vi "InitMiscellaneous.vi"   [LabVIEW 2020]
doc: "This VI initializes miscellaneous devices such as the compressor and any decorations."
uses:
  <vilib>/Rock Robotics/WPI/Compressor/WPI_CompressorFeedbackMode.ctl
  <vilib>/Rock Robotics/SystemInterfaces/DIO/FPGA_DIOPWMChannel.ctl
  refnumbers.vi
  <vilib>/Rock Robotics/WPI/Utilities/WPI_GetSetVariantRefNum.vi
  robotoutputs.vi
types:
  T1 = typedef "FPGA_DIOPWMChannel.ctl" = enum8{"PWM 0", "PWM 1", "PWM 2", "PWM 3", "PWM 4", "PWM 5", "PWM 6", "PWM 7", "PWM 8", "PWM 9", "PWM MXP 0", "PWM MXP 1", "PWM MXP 2", "PWM MXP 3", "PWM MXP 4", "PWM MXP 5", "PWM MXP 6", "PWM MXP 7", "PWM MXP 8", "PWM MXP 9", "Invalid"}
  T2 = typedef "WPI_CompressorFeedbackMode.ctl" = enum16{"Analog Only", "Digital Only", "Hybrid"}
  T3 = cluster{"Feedback Sensor":T2, "Max Pressure (PSI)":dbl, "Min Pressure (PSI)":dbl}
  T4 = typedef "WPI_CompressorDevRef.ctl" = cluster{"DevStatus":errorcluster, "Pneumatics Control Module":u8}
  T5 = typedef "WPI_PWMDeviceRef.ctl" = cluster{"DeviceStatus":errorcluster, "PWM Channel":T1}
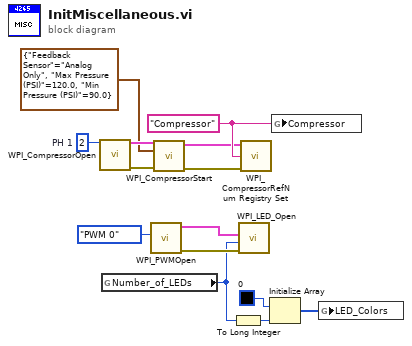
[diagram p0: block diagram]
diagram:
  w11 = "Compressor" ("refnum name")
  w10 = u8 2  # PH 1
  n1 = call <vilib>:"WPI_CompressorOpen.vi"("Pneumatics device (def)"=w10) -> ("CompressorDevRef"=w9:T4, "error out"=w6:errorcluster)  [unwired: 13 in]
  n2 = global read "refnumbers.vi" "Number_of_LEDs"() -> (w1:u16)
  n3 = call <vilib>:"WPI_PWMOpen.vi"("PWM Channel"=FPGA_DIOPWMChannel."PWM 0") -> ("error out"=w3:errorcluster, "PWMDeviceRef"=w4:T5)  [unwired: 9 in]
  n4 = call <vilib>:"WPI_CompressorStart.vi"("error in (no error)"=w6, "Feedback Configuration"=T3 {"Feedback Sensor"=enum."Analog Only", "Max Pressure (PSI)"=120.0, "Min Pressure (PSI)"=90.0}, "CompressorDevRef"=w9) -> ("error out"=w5:errorcluster, "CompressorDevRef"=w7:T4)  [unwired: 7 in]
  n5 = To Long Integer(number=w1) -> (32bit integer=w14:i32)
  n6 = call <vilib>:"WPI_LED_Open.vi"("error in"=w3, "String Length"=w1, "PWMDeviceRef"=w4) -> ()  [unwired: 8 in, 1 out]
  n7 = call <vilib>:"WPI_CompressorRefNum Registry Set.vi"("error in (no error)"=w5, "refnum name"=w11, "CompressorDevRef"=w7) -> ()  [unwired: 7 in, 2 out]
  n8 = Initialize Array(u32 0, w14) -> (w12:u32[])
  n9 = global write "refnumbers.vi" "Compressor"(w11) -> ()
  n10 = global write "robotoutputs.vi" "LED_Colors"(w12) -> ()
